vi "loginjob.vi"() -> ()   [LabVIEW 2012]
panel:
  in  "?":bool
  in  "?":enum32{"calibrate", "test"}(radio)
  in  "PSW:":string
  in  "USER:":string
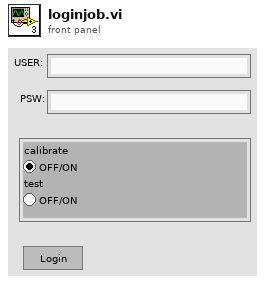
[diagram p1: front panel]
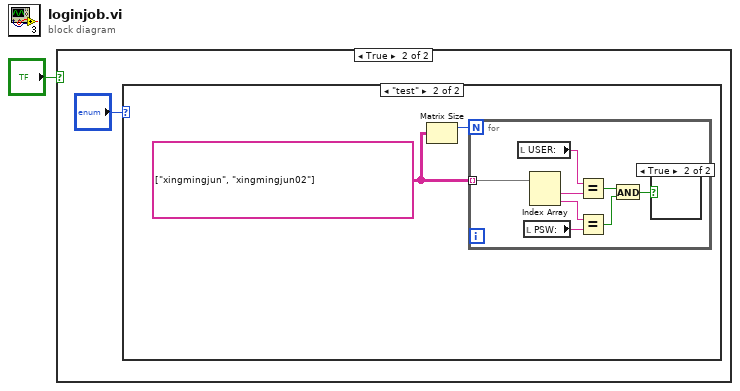
[diagram p0: block diagram]
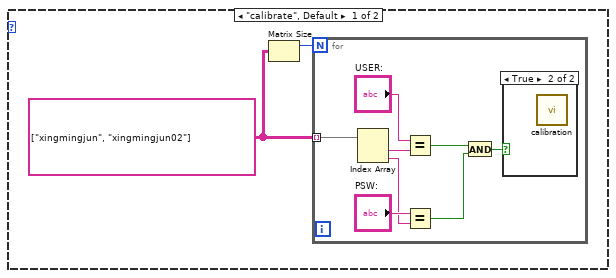
[diagram p3: hidden frame]
diagram:
  n1 = case shown="True" "?" {
    frame False {
    }
    frame True {
      n2 = case shown="\"test\"" "?" {
        frame "calibrate", Default {
          w3 = string[][] [["xingmingjun", "xingmingjun02"]]
          n3 = Matrix Size(0:w3) -> (1:w4:i32)  [unwired: 1 out]
          n4 = for {
            N: w4 -> [_]
            tunnel: w3 -> [w12] mode=indexing
            n5 = Index Array(array=w12) -> (element #1=w10:string, element #2=w8:string)  [unwired: 2 in]
            n6 = Equal?(x="USER:", y=w10) -> (x = y?=w7:bool)
            n7 = Equal?(x="PSW:", y=w8) -> (x = y?=w6:bool)
            n8 = And(x=w7, y=w6) -> (x .and. y?=w5:bool)
            n9 = case shown="True" w5 {
              frame False {
              }
              frame True {
                n10 = call "calibration.vi"() -> ()  [unwired: 12 in]
              }
            }
          }
        }
        frame "test" {
          w13 = string[][] [["xingmingjun", "xingmingjun02"]]
          n11 = Matrix Size(0:w13) -> (1:w14:i32)  [unwired: 1 out]
          n12 = for {
            N: w14 -> [_]
            tunnel: w13 -> [w22] mode=indexing
            n13 = local read "USER:"() -> (w18:string)
            n14 = local read "PSW:"() -> (w20:string)
            n15 = Index Array(array=w22) -> (element #1=w19:string, element #2=w21:string)  [unwired: 2 in]
            n16 = Equal?(x=w18, y=w19) -> (x = y?=w17:bool)
            n17 = Equal?(x=w21, y=w20) -> (x = y?=w16:bool)
            n18 = And(x=w17, y=w16) -> (x .and. y?=w15:bool)
            n19 = case shown="True" w15 {
              frame False {
              }
              frame True {
              }
            }
          }
        }
      }
    }
  }
